vi "Open View.vi"(8 "error in (no error)":errorcluster, 11 "base view in":refnum<class "base view.lvclass">) -> (0 "error out":errorcluster, 3 "base view out":refnum<class "base view.lvclass">)   [LabVIEW 2022 SP3, in "base view.lvclass"]
uses:
  base view.lvclass
  Accessors/Read Events.vi
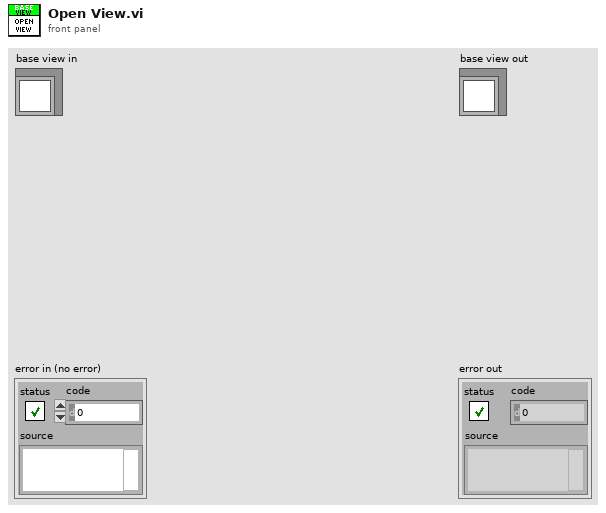
[diagram p1: front panel]
types:
  T1 = typedef "base view.lvclass/Events.ctl" = cluster{"Open":refnum<user-event>, "Close":refnum<user-event>, "Hide":refnum<user-event>}
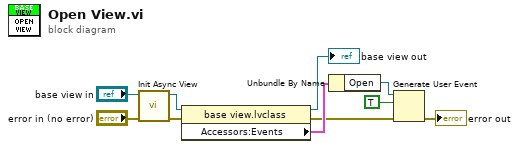
[diagram p0: block diagram]
diagram:
  n1 = call "Init Async View.vi"("error in (no error)"="error in (no error)", "base view in"="base view in") -> ("error out"=w4:errorcluster, "base view out"=w9:refnum<class "base view.lvclass">)  [unwired: 8 in]
  n2 = property class="base view.lvclass"(reference=w9, error in=w4) -> (reference out=→"base view out":refnum<class "base view.lvclass">, error out=w3:errorcluster, "Accessors:Events"=w8:T1)
  n3 = Unbundle By Name(w8) -> ("Open"=w7:refnum<user-event>)
  n4 = Generate User Event(user event=w7, event data cluster=TRUE ("event data"), error in=w3) -> (error out=→"error out":errorcluster)  [unwired: 1 in, 1 out]
